vi "stage-controller.vi"() -> ()   [LabVIEW 2014]
uses:
  Glimpse-master/Microscope plugins/Stage/Move stage command.ctl
  user event out.vi
panel:
  out "Current (X,Y)":cluster{ext[], ext[]}(graph)
  out "At limit 3":bool
  out "At limit 2":bool
  out "At limit":bool
  in  "x,y step (um)":ext=10.0 format="%_5g"
  in  "z step (um)":ext=0.1 format="%_5g"
  out "Current Z (um)":dbl format="%#_13g"
  out "Current Y (um)":dbl format="%#_13g"
  out "Current X (um)":dbl format="%#_13g"
  in  "x-":bool
  in  "y-":bool
  in  "y+":bool
  in  "z-":bool
  in  "z+":bool
  in  "x+":bool
  in  "Reset stage to center\n(x, y, and z)":bool
  in  "Stop":bool
  out "Z Range (mM)":dbl format="%#_13g"
  out "Y Range (mM)":dbl format="%#_13g"
  out "X Range (mM)":dbl format="%#_13g"
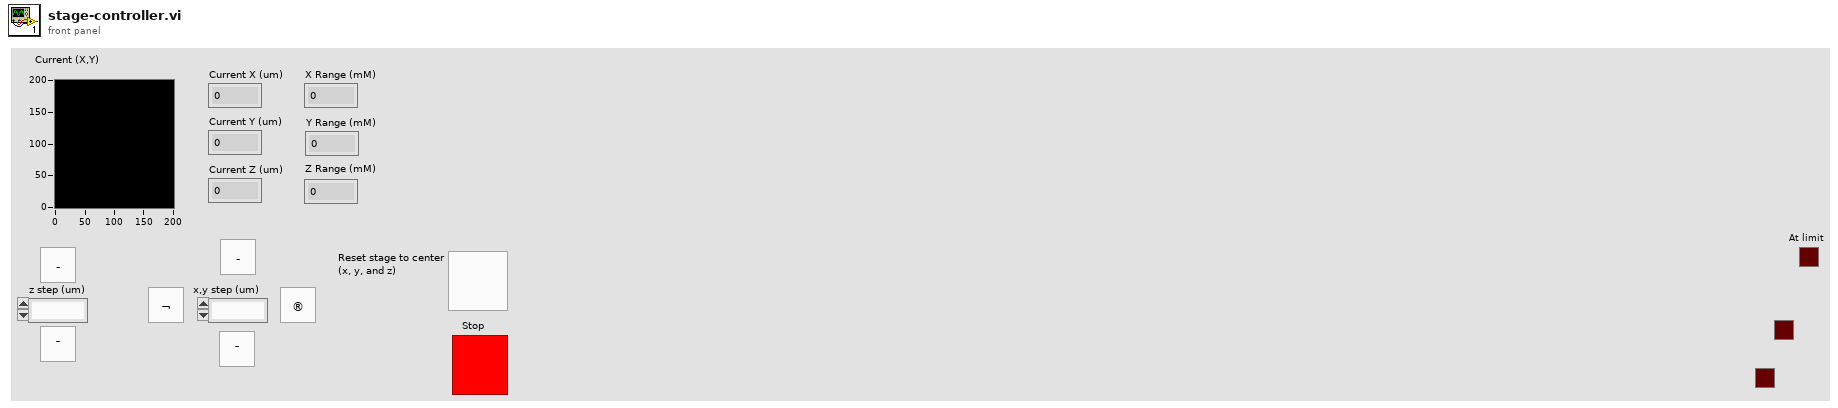
[diagram p1: front panel]
types:
  T1 = cluster{"X Command":dbl, "Y Command":dbl, "Z Command":dbl, "X Position":dbl, "Y Position":dbl, "Z Position":dbl, "X Calibration":dbl, "Y Calibration":dbl, "Z Calibration":dbl}
  T2 = typedef "Move stage command.ctl" = cluster{"dx (um) (0 -> ignore)":ext, "dy (um) (0 -> ignore)":ext, "dz (um) (0 -> ignore)":ext, "Re-center x,y":bool, "Re-center z":bool, "x (um) (-1 -> ignore)":dbl, "y (um) (-1 -> ignore)":dbl, "z (um) (-1 -> ignore)":dbl}
  T3 = cluster{"X Position":dbl, "Y Position":dbl, "Z Position":dbl}
  T4 = cluster{"Current X (um)":ext, "Current Y (um)":ext, "Current Z (um)":ext}
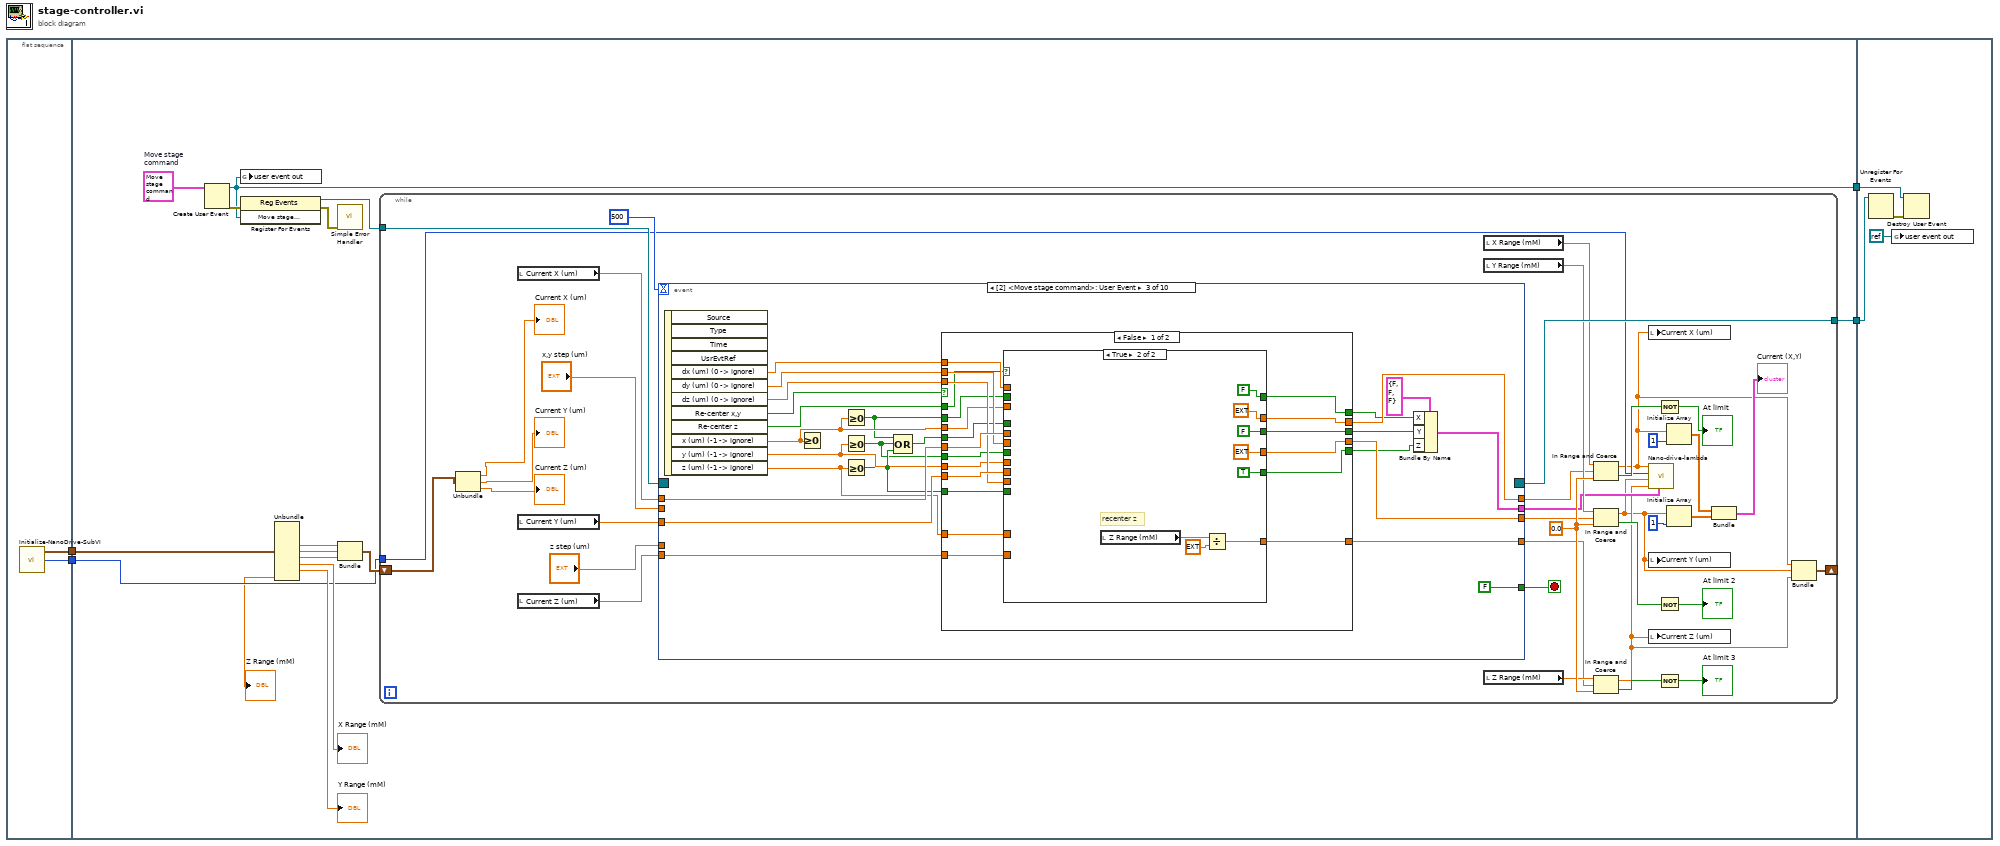
[diagram p0: block diagram]
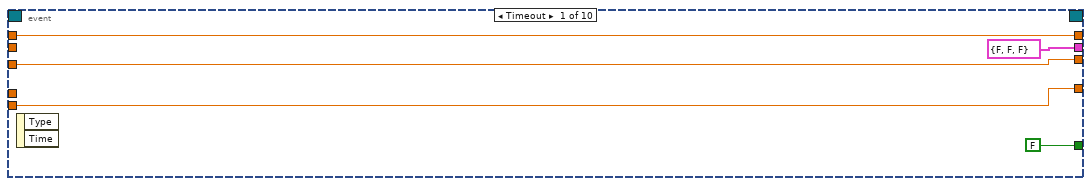
[diagram p2: hidden frame]
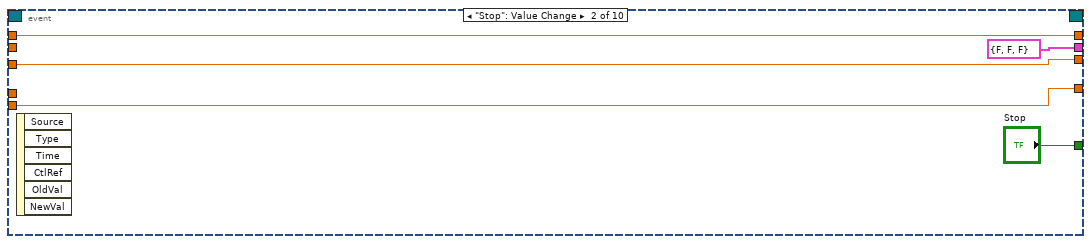
[diagram p3: hidden frame]
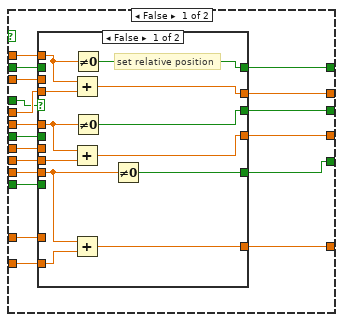
[diagram p4: hidden frame]
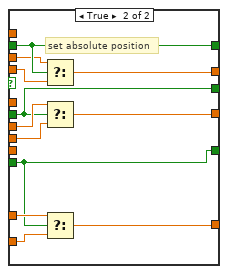
[diagram p5: hidden frame]
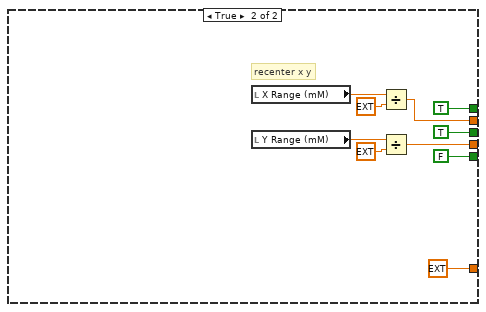
[diagram p6: hidden frame]
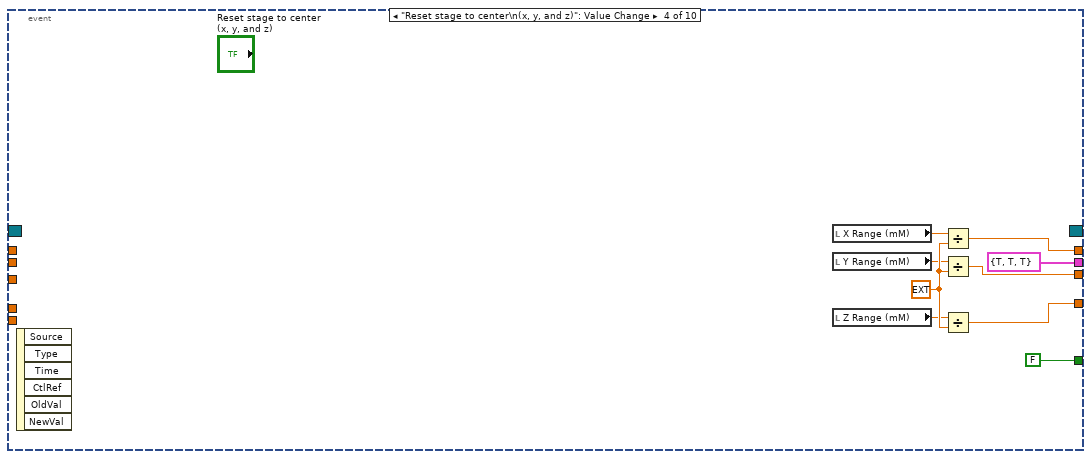
[diagram p7: hidden frame]
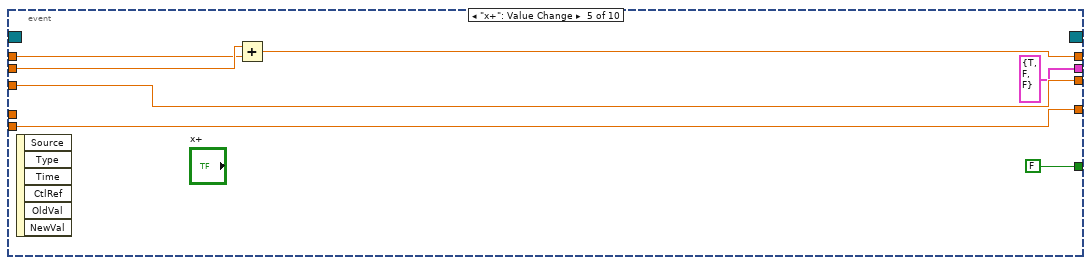
[diagram p8: hidden frame]
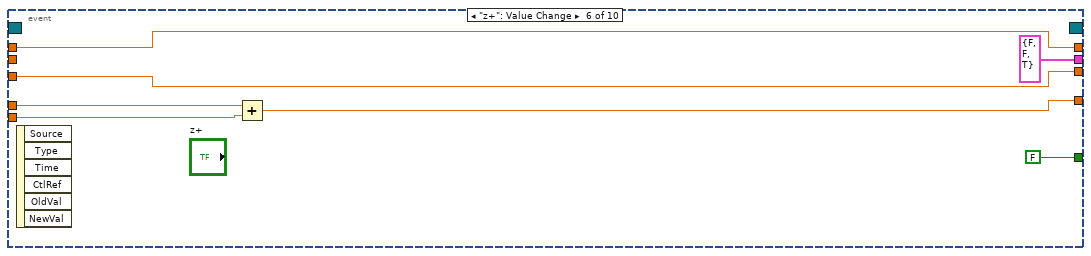
[diagram p9: hidden frame]
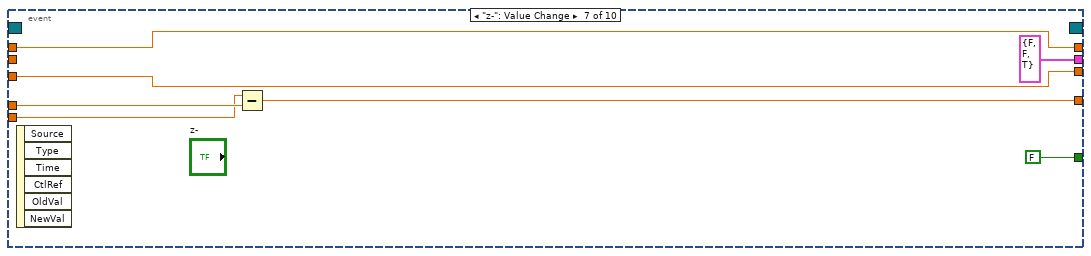
[diagram p10: hidden frame]
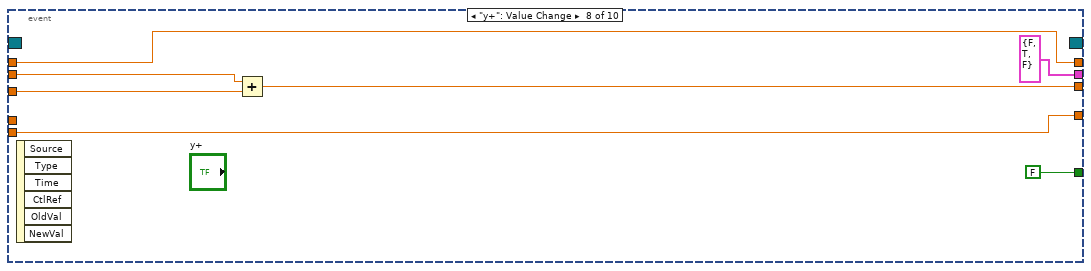
[diagram p11: hidden frame]
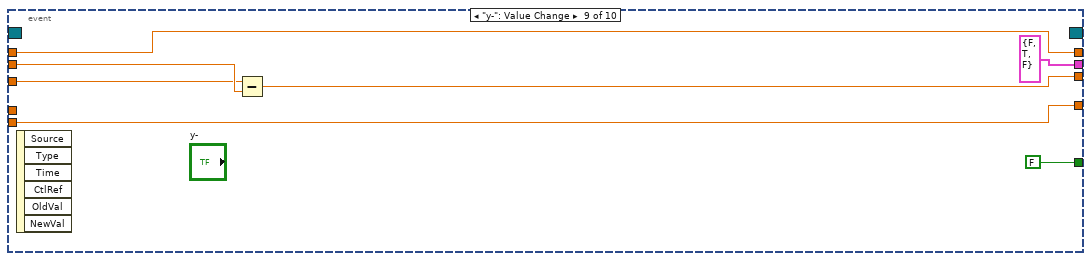
[diagram p12: hidden frame]
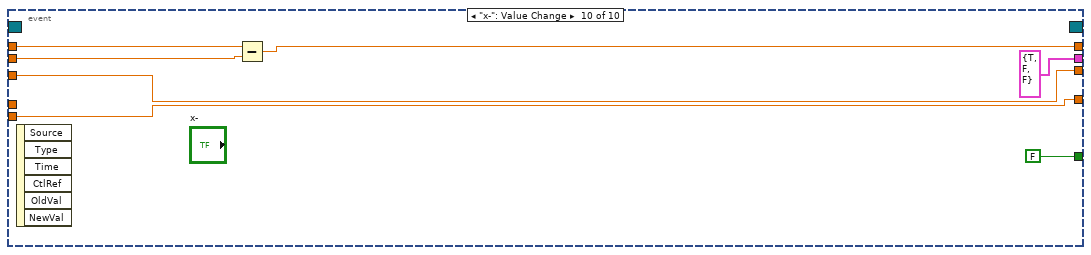
[diagram p13: hidden frame]
diagram:
  n1 = flat-sequence {
    tunnel: [w6] -> w4
    tunnel: [w5] -> w1
    tunnel: w4 -> [w21]
    tunnel: [w10] -> w3
    tunnel: [w9] -> w2
    tunnel: w1 -> [w8]
    tunnel: w3 -> [w227]
    tunnel: w2 -> [w226]
    frame #0 {
      n2 = call "Initialize-NanoDrive-SubVI.vi"() -> ("Output Pos Info"=w6:T1, "Handle"=w5:i32)  [unwired: 1 in, 1 out]
    }
    frame #1 {
      w17 = T2 {"dx (um) (0 -> ignore)"=0.0, "dy (um) (0 -> ignore)"=0.0, "dz (um) (0 -> ignore)"=0.0, "Re-center x,y"=FALSE, "Re-center z"=FALSE, "x (um) (-1 -> ignore)"=-1.0, "y (um) (-1 -> ignore)"=-1.0, "z (um) (-1 -> ignore)"=-1.0}  # Move stage command
      n3 = Create User Event(user event datatype=w17) -> (user event=w9:refnum<user-event>, error out=w12:errorcluster)  [unwired: 1 in]
      n4 = global write "user event out.vi" "user event out"(w9) -> ()
      n5 = register-events(error in=w12, w9) -> (reference out=w11:refnum<event-registration>, error out=w13:errorcluster)  [unwired: 1 in]
      n6 = Unbundle(w21) -> ("X Position"=w20:dbl, "Y Position"=w19:dbl, "Z Position"=w18:dbl, "X Calibration"=→"X Range (mM)":dbl, "Y Calibration"=→"Y Range (mM)":dbl, "Z Calibration"=→"Z Range (mM)":dbl)  [unwired: 3 out]
      n7 = call <vilib>:"Simple Error Handler.vi"("error in (no error)"=w13) -> ()  [unwired: 1 in, 8 out]
      n8 = Bundle("X Position"=w20, "Y Position"=w19, "Z Position"=w18) -> (w14:T3)  [unwired: 1 in]
      n9 = while {
        shift-right: [w26] -> _
        shift-left: w14 -> [w25]
        tunnel: w11 -> [w52]
        tunnel: [w51] -> w10
        tunnel: w8 -> [w30]
        stop <- w53 stop-if-true
        w50 = 0.0
        n10 = Unbundle(w25) -> ("Current X (um)"=→"Current X (um)":ext, "Current Y (um)"=→"Current Y (um)":ext, "Current Z (um)"=→"Current Z (um)":ext)
        n11 = local read "Current X (um)"() -> (w57:dbl)
        n12 = local read "Current Y (um)"() -> (w58:dbl)
        n13 = local read "Current Z (um)"() -> (w56:dbl)
        n14 = event shown="[2] <Move stage\ncommand>: User Event" {
          selector: w52 -> [_ _ _ _ _ _ _ _ _ _]
          dyn-events: [_ _ _ _ _ _ _ _ _ _] -> w51
          timeout: 500 -> [_ _ _ _ _ _ _ _ _ _]
          tunnel: [FALSE ("Stop") "Stop" FALSE ("Stop") FALSE ("Stop") FALSE ("Stop") FALSE ("Stop") FALSE ("Stop") FALSE ("Stop") FALSE ("Stop") FALSE ("Stop")] -> w53
          tunnel: w57 -> [w62 w67 w92 _ w186 w195 w201 w205 w214 w221]
          tunnel: w58 -> [w61 w66 w91 _ w185 w190 w200 w207 w211 w220]
          tunnel: w56 -> [w60 w65 w90 _ w184 w192 w197 w209 w215 w219]
          tunnel: [w62 w67 w87 w177 w188 w195 w201 w205 w214 w223] -> w46
          tunnel: [w61 w66 w88 w180 w185 w190 w200 w208 w216 w220] -> w45
          tunnel: [w60 w65 w89 w179 w184 w194 w203 w209 w215 w219] -> w44
          tunnel: [cluster{"X":bool, "Y":bool, "Z":bool} {"X"=FALSE, "Y"=FALSE, "Z"=FALSE} ("Set this axis?") cluster{"X":bool, "Y":bool, "Z":bool} {"X"=FALSE, "Y"=FALSE, "Z"=FALSE} ("Set this axis?") w80 cluster{"X":bool, "Y":bool, "Z":bool} {"X"=TRUE, "Y"=TRUE, "Z"=TRUE} ("Set this axis?") cluster{"X":bool, "Y":bool, "Z":bool} {"X"=TRUE, "Y"=FALSE, "Z"=FALSE} ("Set this axis?") cluster{"X":bool, "Y":bool, "Z":bool} {"X"=FALSE, "Y"=FALSE, "Z"=TRUE} ("Set this axis?") cluster{"X":bool, "Y":bool, "Z":bool} {"X"=FALSE, "Y"=FALSE, "Z"=TRUE} ("Set this axis?") cluster{"X":bool, "Y":bool, "Z":bool} {"X"=FALSE, "Y"=TRUE, "Z"=FALSE} ("Set this axis?") cluster{"X":bool, "Y":bool, "Z":bool} {"X"=FALSE, "Y"=TRUE, "Z"=FALSE} ("Set this axis?") cluster{"X":bool, "Y":bool, "Z":bool} {"X"=TRUE, "Y"=FALSE, "Z"=FALSE} ("Set this axis?")] -> w31
          tunnel: "x,y step (um)" -> [_ _ _ _ w187 _ _ w206 w212 w222]
          tunnel: "z step (um)" -> [_ _ _ _ _ w191 w198 _ _ _]
          event Timeout {
            n15 = event-data() -> ()  [unwired: 3 out]
          }
          event "Stop": Value Change {
            n16 = event-data() -> ()  [unwired: 7 out]
          }
          event User Event {
            n17 = event-data() -> ("dx (um) (0 -> ignore)"=w85:ext, "dy (um) (0 -> ignore)"=w84:ext, "dz (um) (0 -> ignore)"=w83:ext, "Re-center x,y"=w82:bool, "Re-center z"=w76:bool, "x (um) (-1 -> ignore)"=w72:dbl, "y (um) (-1 -> ignore)"=w73:dbl, "z (um) (-1 -> ignore)"=w74:dbl)  [unwired: 5 out]
            n18 = Greater Or Equal To 0?(x=w72) -> ()  [unwired: 1 out]
            n19 = Greater Or Equal To 0?(x=w72) -> (x >= 0?=w69:bool)
            n20 = Greater Or Equal To 0?(x=w73) -> (x >= 0?=w70:bool)
            n21 = Greater Or Equal To 0?(x=w74) -> (x >= 0?=w71:bool)
            n22 = Compound Arithmetic op=OR(w69, w70, w71) -> (w75:bool)
            n23 = case shown="False" w82 {
              tunnel: w92 -> [w112 _]
              tunnel: w91 -> [w111 _]
              tunnel: w90 -> [w110 _]
              tunnel: [w109 ext 0.0] -> w89
              tunnel: [w108 w166] -> w88
              tunnel: [w107 w168] -> w87
              tunnel: w85 -> [w106 _]
              tunnel: w84 -> [w105 _]
              tunnel: w83 -> [w104 _]
              tunnel: [w103 FALSE] -> w79
              tunnel: [w102 TRUE] -> w78
              tunnel: [w101 TRUE] -> w77
              tunnel: w76 -> [w100 _]
              tunnel: w75 -> [w99 _]
              tunnel: w74 -> [w98 _]
              tunnel: w73 -> [w97 _]
              tunnel: w72 -> [w96 _]
              tunnel: w71 -> [w95 _]
              tunnel: w70 -> [w94 _]
              tunnel: w69 -> [w93 _]
              frame False {
                n24 = case shown="True" w100 {
                  tunnel: w112 -> [w131 _]
                  tunnel: w111 -> [w130 _]
                  tunnel: w110 -> [w129 _]
                  tunnel: [w128 w162] -> w109
                  tunnel: [w127 ext 0.0] -> w108
                  tunnel: [w126 ext 0.0] -> w107
                  tunnel: w106 -> [w125 _]
                  tunnel: w105 -> [w124 _]
                  tunnel: w104 -> [w123 _]
                  tunnel: [w122 TRUE] -> w103
                  tunnel: [w121 FALSE] -> w102
                  tunnel: [w120 FALSE] -> w101
                  tunnel: w99 -> [w119 _]
                  tunnel: w98 -> [w118 _]
                  tunnel: w97 -> [w117 _]
                  tunnel: w96 -> [w116 _]
                  tunnel: w95 -> [w115 _]
                  tunnel: w94 -> [w114 _]
                  tunnel: w93 -> [w113 _]
                  frame False {
                    n25 = case shown="False" w119 {
                      tunnel: w131 -> [w143 w151]
                      tunnel: w130 -> [w142 w148]
                      tunnel: w129 -> [w141 w145]
                      tunnel: [w140 w147] -> w128
                      tunnel: [w139 w150] -> w127
                      tunnel: [w138 w154] -> w126
                      tunnel: w125 -> [w137 _]
                      tunnel: w124 -> [w136 _]
                      tunnel: w123 -> [w135 _]
                      tunnel: [w134 w144] -> w122
                      tunnel: [w133 w149] -> w121
                      tunnel: [w132 w153] -> w120
                      tunnel: w118 -> [_ w146]
                      tunnel: w117 -> [_ w155]
                      tunnel: w116 -> [_ w152]
                      tunnel: w115 -> [_ w144]
                      tunnel: w114 -> [_ w149]
                      tunnel: w113 -> [_ w153]
                      frame False {
                        # "set relative position"
                        n26 = Add(x=w137, y=w143) -> (x+y=w138:ext)
                        n27 = Add(x=w136, y=w142) -> (x+y=w139:ext)
                        n28 = Add(x=w135, y=w141) -> (x+y=w140:ext)
                        n29 = Not Equal To 0?(x=w137) -> (x != 0?=w132:bool)
                        n30 = Not Equal To 0?(x=w136) -> (x != 0?=w133:bool)
                        n31 = Not Equal To 0?(x=w135) -> (x != 0?=w134:bool)
                      }
                      frame True {
                        # "set absolute position"
                        n32 = Select(t=w152, s=w153, f=w151) -> (s? t:f=w154:dbl)
                        n33 = Select(t=w155, s=w149, f=w148) -> (s? t:f=w150:dbl)
                        n34 = Select(t=w146, s=w144, f=w145) -> (s? t:f=w147:dbl)
                      }
                    }
                  }
                  frame True {
                    # "recenter z"
                    n35 = local read "Z Range (mM)"() -> (w156:dbl)
                    n36 = Divide(x=w156, y=ext 2.0) -> (x/y=w162:ext)
                  }
                }
              }
              frame True {
                # "recenter x y"
                n37 = local read "X Range (mM)"() -> (w165:dbl)
                n38 = local read "Y Range (mM)"() -> (w164:dbl)
                n39 = Divide(x=w165, y=ext 2.0) -> (x/y=w168:ext)
                n40 = Divide(x=w164, y=ext 2.0) -> (x/y=w166:ext)
              }
            }
            n41 = Bundle By Name(cluster=cluster{"X":bool, "Y":bool, "Z":bool} {"X"=FALSE, "Y"=FALSE, "Z"=FALSE} ("Set this axis?"), "X"=w77, "Y"=w78, "Z"=w79) -> (w80:cluster{"X":bool, "Y":bool, "Z":bool})
          }
          event "Reset stage to center\n(x, y, and z)": Value Change {
            w178 = ext 2.0 ("y")
            n42 = event-data() -> ()  [unwired: 7 out]
            n43 = local read "X Range (mM)"() -> (w174:dbl)
            n44 = local read "Y Range (mM)"() -> (w175:dbl)
            n45 = local read "Z Range (mM)"() -> (w176:dbl)
            n46 = Divide(x=w174, y=w178) -> (x/y=w177:ext)
            n47 = Divide(x=w175, y=w178) -> (x/y=w180:ext)
            n48 = Divide(x=w176, y=w178) -> (x/y=w179:ext)
          }
          event "x+": Value Change {
            n49 = event-data() -> ()  [unwired: 7 out]
            n50 = Add(x=w187, y=w186) -> (x+y=w188:ext)
          }
          event "z+": Value Change {
            n51 = event-data() -> ()  [unwired: 7 out]
            n52 = Add(x=w191, y=w192) -> (x+y=w194:ext)
          }
          event "z-": Value Change {
            n53 = event-data() -> ()  [unwired: 7 out]
            n54 = Subtract(x=w197, y=w198) -> (x-y=w203:ext)
          }
          event "y+": Value Change {
            n55 = event-data() -> ()  [unwired: 7 out]
            n56 = Add(x=w206, y=w207) -> (x+y=w208:ext)
          }
          event "y-": Value Change {
            n57 = event-data() -> ()  [unwired: 7 out]
            n58 = Subtract(x=w211, y=w212) -> (x-y=w216:ext)
          }
          event "x-": Value Change {
            n59 = event-data() -> ()  [unwired: 7 out]
            n60 = Subtract(x=w221, y=w222) -> (x-y=w223:ext)
          }
        }
        n61 = local read "X Range (mM)"() -> (w48:dbl)
        n62 = local read "Y Range (mM)"() -> (w49:dbl)
        n63 = local read "Z Range (mM)"() -> (w47:dbl)
        n64 = In Range and Coerce(upper limit=w48, x=w46, lower limit=w50) -> (coerced(x)=w27:ext, In Range?=w42:bool)
        n65 = In Range and Coerce(upper limit=w49, x=w45, lower limit=w50) -> (coerced(x)=w28:ext, In Range?=w40:bool)
        n66 = In Range and Coerce(upper limit=w47, x=w44, lower limit=w50) -> (coerced(x)=w29:ext, In Range?=w38:bool)
        n67 = local write "Current X (um)"(w27) -> ()
        n68 = call "Nano-drive-lambda.vi"("Set this axis?"=w31, "Z (um)"=w29, "Y (um)"=w28, "Numeric"=w30, "X (um)"=w27) -> ()  [unwired: 6 in]
        n69 = local write "Current Y (um)"(w28) -> ()
        n70 = local write "Current Z (um)"(w29) -> ()
        n71 = Not(x=w42) -> (.not. x?=→"At limit":bool)
        n72 = Not(x=w40) -> (.not. x?=→"At limit 2":bool)
        n73 = Not(x=w38) -> (.not. x?=→"At limit 3":bool)
        n74 = Initialize Array(w27, 1) -> (w34:ext[])
        n75 = Initialize Array(w28, 1) -> (w33:ext[])
        n76 = Bundle(w34, w33) -> (→"Current (X,Y)":cluster{ext[], ext[]})  [unwired: 1 out]
        n77 = Bundle("Current X (um)"=w27, "Current Y (um)"=w28, "Current Z (um)"=w29) -> (w26:T4)  [unwired: 1 in]
      }
    }
    frame #2 {
      n78 = Unregister For Events(event registration refnum=w227) -> (error out=w228:errorcluster)  [unwired: 1 in]
      n79 = global write "user event out.vi" "user event out"(refnum<k0> refnum) -> ()
      n80 = Destroy User Event(user event=w226, error in=w228) -> ()  [unwired: 1 out]
    }
  }
